vi "eraseCI1_img.vi"   [LabVIEW 2013]
types:
  T1 = cluster{" CI1":refnum<k21>, "E_CI1":errorcluster}
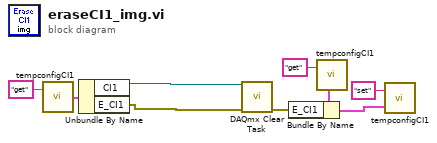
[diagram p0: block diagram]
diagram:
  n1 = call "tempconfigCI1.vi"("command"="get") -> ("Temp Config out"=w8:T1)  [unwired: 1 in]
  n2 = Unbundle By Name(w8) -> ("CI1"=w2:refnum<k21>, "E_CI1"=w1:errorcluster)
  n3 = call <vilib>:"DAQmx Clear Task.vi"("task in"=w2, "error in"=w1) -> ("error out"=w4:errorcluster)  [unwired: 13 in]
  n4 = call "tempconfigCI1.vi"("command"="get") -> ("Temp Config out"=w5:T1)  [unwired: 1 in]
  n5 = Bundle By Name(cluster=w5, "E_CI1"=w4) -> (w3:T1)
  n6 = call "tempconfigCI1.vi"("Temp Config in"=w3, "command"="set") -> ()  [unwired: 1 out]
